vi "SP Sort Adapters by Port.vi"(1 "Adapters":T1[](array[typedef])) -> (0 "Sorted Adapters":T1[](array[typedef]))   [LabVIEW 2011]
uses:
  TypeDefs/SP Adapter.ctl
  TypeDefs/SP Data.ctl
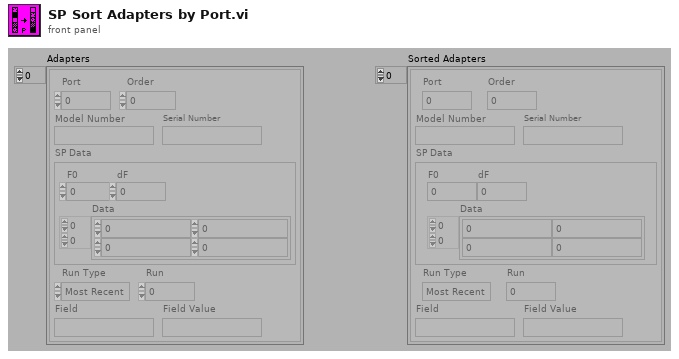
[diagram p1: front panel]
types:
  T1 = typedef "SP Adapter.ctl" = cluster{"Port":i8, "Order":i8, "Model Number":string, "Serial Number":string, "SP Data":T2, "Run Type":enum16{"Most Recent", "Run #", "Match Field"}, "Run":i32, "Field":string, "Field Value":string}
  T2 = typedef "SP Data.ctl" = cluster{"F0":dbl, "dF":dbl, "Data":cdb[][]}
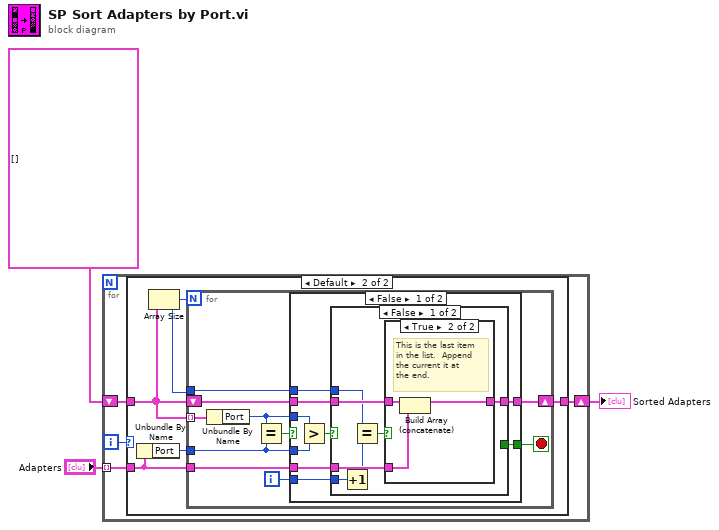
[diagram p0: block diagram]
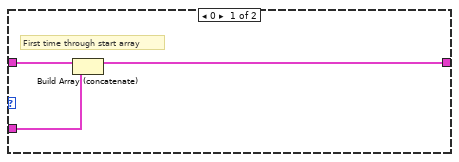
[diagram p2: hidden frame]
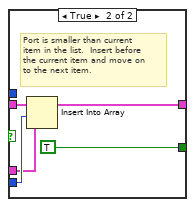
[diagram p4: hidden frame]
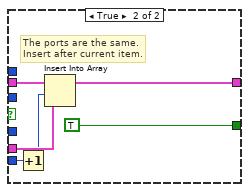
[diagram p5: hidden frame]
diagram:
  n1 = for {
    tunnel: "Adapters" -> [w6] mode=indexing
    shift-right: [w4] -> w1
    shift-left: T1[] [] ("Adapters") -> [w5]
    i -> [w7]
    n2 = case shown="Default" w7 {
      tunnel: w6 -> [w8 w15]
      tunnel: w5 -> [w10 w12]
      tunnel: [w9 w14] -> w4
      frame 0 {
        # "First time through start array"
        n3 = Build Array (concatenate)(w10, w8) -> (w9:T1[])
      }
      frame Default {
        n4 = Unbundle By Name(w15) -> ("Port"=w13:i8)
        n5 = Array Size(array=w12) -> (size(s)=w11:i32)
        n6 = for {
          N: w11 -> [_]
          tunnel: w12 -> [w25] mode=indexing
          tunnel: w13 -> [w23]
          shift-right: [w20] -> w14
          shift-left: w12 -> [w22]
          tunnel: w15 -> [w21]
          tunnel: w11 -> [w17]
          i -> [w19]
          stop <- w18 stop-if-true
          n7 = Unbundle By Name(w25) -> ("Port"=w16:i8)
          n8 = Equal?(x=w16, y=w23) -> (x = y?=w24:bool)
          n9 = case shown="False" w24 {
            tunnel: w16 -> [w34 _]
            tunnel: w23 -> [w33 _]
            tunnel: w22 -> [w31 w56]
            tunnel: w21 -> [w30 w55]
            tunnel: [w29 w52] -> w20
            tunnel: w19 -> [w28 w54]
            tunnel: [w27 TRUE] -> w18
            tunnel: w17 -> [w26 _]
            frame False {
              n10 = Greater?(x=w34, y=w33) -> (0:w32:bool)
              n11 = case shown="False" w32 {
                tunnel: w31 -> [w41 w50]
                tunnel: w30 -> [w40 w47]
                tunnel: [w35 w49] -> w29
                tunnel: w28 -> [w39 w48]
                tunnel: [_ TRUE] -> w27
                tunnel: w26 -> [w36 _]
                frame False {
                  n12 = Increment(x=w39) -> (x+1=w37:i32)
                  n13 = Equal?(x=w36, y=w37) -> (x = y?=w38:bool)
                  n14 = case shown="True" w38 {
                    tunnel: w41 -> [w42 w45]
                    tunnel: w40 -> [_ w44]
                    tunnel: [w42 w43] -> w35
                    frame False {
                      # "Move on to the\nnext item and\ncheck again."
                    }
                    frame True {
                      # "This is the last item\nin the list.  Append\nthe current it at \nthe end."
                      n15 = Build Array (concatenate)(w45, w44) -> (w43:T1[])
                    }
                  }
                }
                frame True {
                  # "Port is smaller than current\nitem in the list.  Insert before\nthe current item and move on\nto the next item."
                  n16 = Insert Into Array(array=w50, index=w48, new element=w47) -> (w49:T1[])
                }
              }
            }
            frame True {
              # "The ports are the same.\nInsert after current item."
              n17 = Increment(x=w54) -> (x+1=w53:i32)
              n18 = Insert Into Array(array=w56, index=w53, new element=w55) -> (w52:T1[])
            }
          }
        }
      }
    }
  }
  "Sorted Adapters" <- w1
